vi "Add Actor Message.vi"(6 "Mouse Position":T1 caption="鼠标位置", 7 "User VI Ref":refnum<vi> caption="用户VI引用", 8 "Is Multi-select?":bool caption="为多选？", 9 "Remaining Items":refnum<vi>[](array[refnum]) caption="剩余项", 10 "Affected Items":T8 caption="受影响的项", 11 "Menu Refnum":refnum<k9> caption="菜单引用句柄") -> (3 "Menu Items To Add":T2[](array[typedef]) caption="待添加菜单项")   [LabVIEW 2020]
doc: "该VI属于修改LabVIEW快捷菜单部分。这是创建快捷菜单时调用的生成VI。该VI为LabVIEW输入添加到菜单的快捷菜单项。"
uses:
  <resource>/plugins/PopupMenus/support/Shortcut Menu Item Definition.ctl
  <resource>/plugins/PopupMenus/support/Transaction Control.ctl
  <resource>/plugins/PopupMenus/support/Position In Menu.ctl
  <resource>/plugins/PopupMenus/support/Relative Position.ctl
  <resource>/plugins/PopupMenus/support/Checkmark Status.ctl
  <resource>/plugins/PopupMenus/support/Enabled Menu Item Status.ctl
  Add Actor Message.ctl
  <vilib>/Utility/miscctls.llb/LVPositionTypeDef.ctl
  <vilib>/Utility/Data Type/NI_Data Type.lvlib
panel:
  # "弹出插件时必须遵循的规则：\n*该VI的文件名称必须与LLB的文件名称匹配－不同的只是文件扩展名。\n*VI必须禁用调试，否则它将作为插件被忽略。\n*所有菜单项的“标签后缀 + VI文件名”必须少于240个字符。\n*可从自定义类型断开连接“受影响的项”，从而加快插件的加载速度。存在该自定义类型的目的是使该VI和执行VI使用相同的类型。\n*除“受影响的项”之外，前面板上的其他所有控件都已锁定，以防被意外编辑。除“受影响的项”簇中的元素外，不要修改控件的类型或名称。\n*请参考即时帮助，了解每个控件的详细信息。"
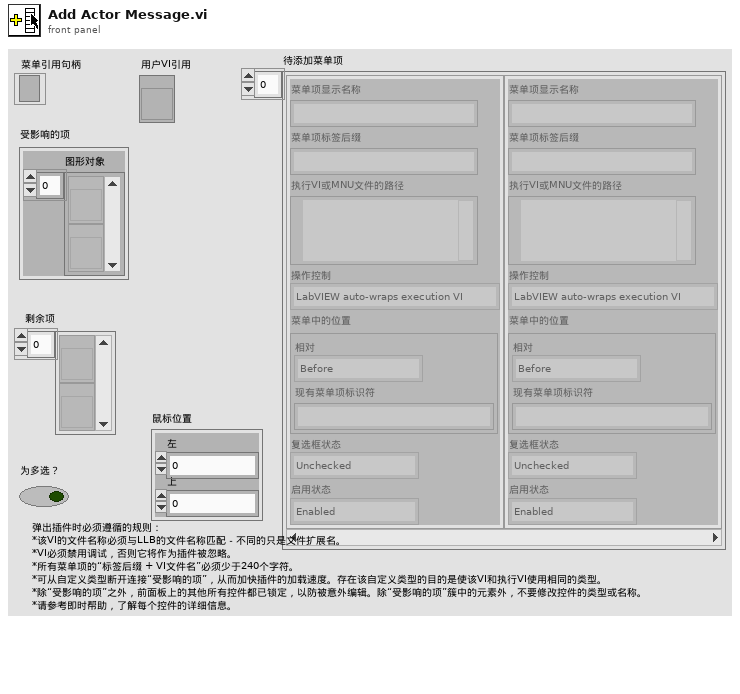
[diagram p1: front panel]
types:
  T1 = typedef "LVPositionTypeDef.ctl" = cluster{"Left":i32, "Top":i32}
  T2 = typedef "Shortcut Menu Item Definition.ctl" = cluster{"Menu Item Display Name":string, "Menu Item Tag Suffix":string, "Path To Execution VI or MNU":path, "Transaction Control":T3, "Position In Menu":T4, "Checkmark Status":T6, "Enabled Status":T7}
  T3 = typedef "Transaction Control.ctl" = enum8{"LabVIEW auto-wraps execution VI", "Execution VI will define if needed"}
  T4 = typedef "Position In Menu.ctl" = cluster{"Relative":T5, "Existing Item Tag":string}
  T5 = typedef "Relative Position.ctl" = enum8{"Before", "Instead of", "After", "Into Submenu"}
  T6 = typedef "Checkmark Status.ctl" = enum8{"Unchecked", "Checked"}
  T7 = typedef "Enabled Menu Item Status.ctl" = enum8{"Enabled", "Disabled"}
  T8 = typedef "Add Actor Message.ctl" = cluster{"GObj":refnum<vi>[]}
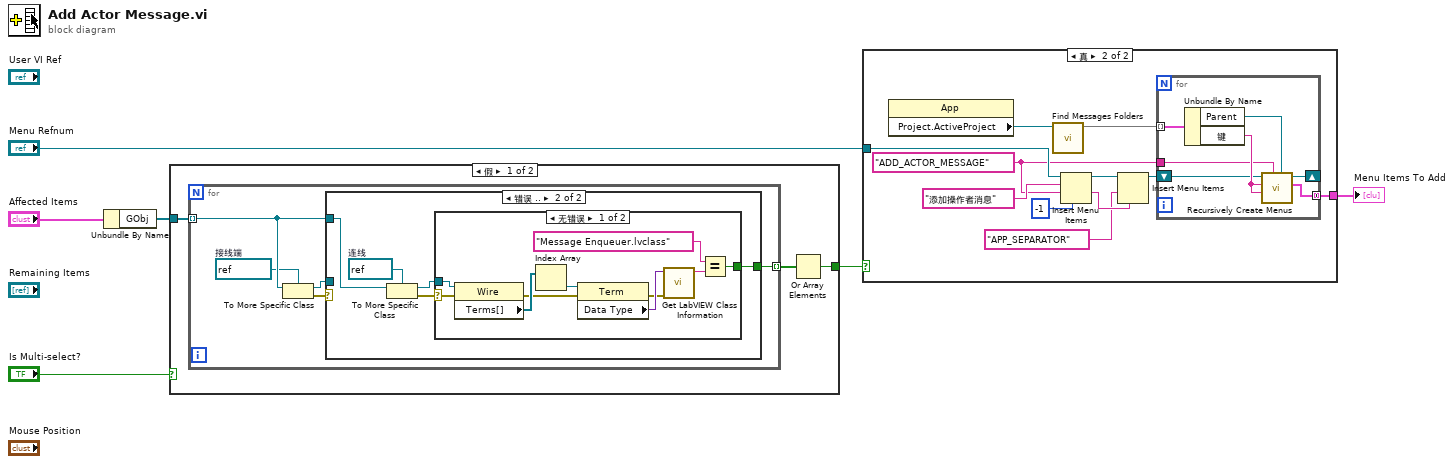
[diagram p0: block diagram]
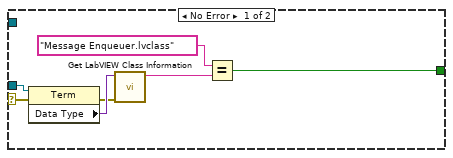
[diagram p2: hidden frame]
diagram:
  n1 = Unbundle By Name("Affected Items") -> ("GObj"=w1:refnum<vi>[])
  n2 = case shown="假" "Is Multi-select?" {
    tunnel: [w7 _] -> w2
    tunnel: w1 -> [w8 _]
    frame False {
      n3 = for {
        tunnel: [w14] -> w9 mode=indexing
        tunnel: w8 -> [w13] mode=indexing
        w11 = refnum<vi> refnum  # 接线端
        n4 = To More Specific Class(target class=w11, reference=w13) -> (specific class reference=w12:refnum<vi>, error out=w10:errorcluster)  [unwired: 1 in]
        n5 = case shown="错误 .." w10 {
          selector: w10 -> [w20 _]
          tunnel: w12 -> [w21 _]
          tunnel: w13 -> [_ w25]
          tunnel: [w16 w22] -> w14
          frame No Error {
            n6 = property class="Term"(reference=w21, error in=w20) -> (error out=w18:errorcluster, "Data Type"=w19:variant)  [unwired: 1 out]
            n7 = call <vilib>:"Get LabVIEW Class Information.vi"("error in (no error)"=w18, "variant"=w19) -> ("LabVIEW class file name"=w15:string)  [unwired: 7 in, 2 out]
            n8 = Equal?(x="Message Enqueuer.lvclass" ("y"), y=w15) -> (x = y?=w16:bool)
          }
          frame Error {
            w26 = refnum<vi> refnum  # 连线
            n9 = To More Specific Class(target class=w26, reference=w25) -> (specific class reference=w24:refnum<vi>, error out=w23:errorcluster)  [unwired: 1 in]
            n10 = case shown="无错误" w23 {
              selector: w23 -> [w32 _]
              tunnel: w24 -> [w33 _]
              tunnel: [w27 _] -> w22
              frame No Error {
                n11 = property class="Wire"(reference=w33, error in=w32) -> (error out=w31:errorcluster, "Terms[]"=w35:refnum<vi>[])  [unwired: 1 out]
                n12 = Index Array(array=w35) -> (element=w34:refnum<vi>)  [unwired: 1 in]
                n13 = property class="Term"(reference=w34, error in=w31) -> (error out=w30:errorcluster, "Data Type"=w36:variant)  [unwired: 1 out]
                n14 = call <vilib>:"Get LabVIEW Class Information.vi"("error in (no error)"=w30, "variant"=w36) -> ("LabVIEW class file name"=w29:string)  [unwired: 7 in, 2 out]
                n15 = Equal?(x="Message Enqueuer.lvclass" ("y"), y=w29) -> (x = y?=w27:bool)
              }
              frame Error {
              }
            }
          }
        }
      }
      n16 = Or Array Elements(Boolean array=w9) -> (logical OR=w7:bool)
    }
    frame True {
    }
  }
  n17 = case shown="真" w2 {
    tunnel: "Menu Refnum" -> [_ w47]
    tunnel: [_ w43] -> w5
    frame False {
    }
    frame True {
      w39 = "ADD_ACTOR_MESSAGE" ("项标识符")
      n18 = property class="App"() -> ("Project.ActiveProject"=w41:refnum<vi>)  [unwired: 2 in, 2 out]
      n19 = call "Find Messages Folders.vi"("项目输入"=w41) -> ("Messages Folders"=w42:map{string, refnum<vi>})  [unwired: 9 in, 1 out]
      n20 = Insert Menu Items(4:-1, 7:w39, 8:"添加操作者消息", 9:w47) -> (1:w38:string, 3:w44:refnum<k9>)  [unwired: 2 in, 1 out]
      n21 = Insert Menu Items(4:w38, 7:"APP_SEPARATOR", 9:w44) -> (3:w40:refnum<k9>)  [unwired: 3 in, 2 out]
      n22 = for {
        tunnel: w42 -> [w54] mode=indexing
        tunnel: w39 -> [w52]
        shift-right: [w50] -> _
        shift-left: w40 -> [w51]
        tunnel: [w49] -> w43 mode=concatenating
        n23 = Unbundle By Name(w54) -> ("Parent"=w48:refnum<vi>, "键"=w53:string)
        n24 = call "Recursively Create Menus.vi"("Parent"=w48, "菜单标识符"=w52, "项标识符"=w53, "项名称"=w53, "菜单引用 in"=w51) -> ("Menu Items To Add"=w49:T2[], "菜单引用 out"=w50:refnum<k9>)  [unwired: 4 in, 1 out]
      }
    }
  }
  "Menu Items To Add" <- w5
